vi "Write_parameter.vi"(8 "error in (no error)":errorcluster caption="entrée d'erreur (pas d'erreur)", 10 "Parameter":string, 11 "Class DIO en entrée":refnum<class "Class Instrument Ana.lvclass">) -> (0 "error out":errorcluster caption="sortie d'erreur", 3 "Class DIO en Sortie":refnum<class "Class Instrument Ana.lvclass">)   [LabVIEW 2020, in "Library Instrument & Equipement.lvlib" / "Library Instruments.lvlib" / "Class Instrument Ana.lvclass"]
uses:
  Class Instrument Ana.lvclass
  Ana/Class Ana (Default)/Class Ana (Default).lvclass
  JSON API/JSON Value/Set from JSON string.vi
  Instrument (Default)/Class Instrument (Default).lvclass
  JSON API/JSON Value/JSON Value.lvclass
  Class Instrument Ana.lvclass/Class Instrument Ana.ctl
  JSON API/Variant JSON/Variant JSON.lvlib
  JSON API/Get Polymorphic/JSON GetSet.lvlib
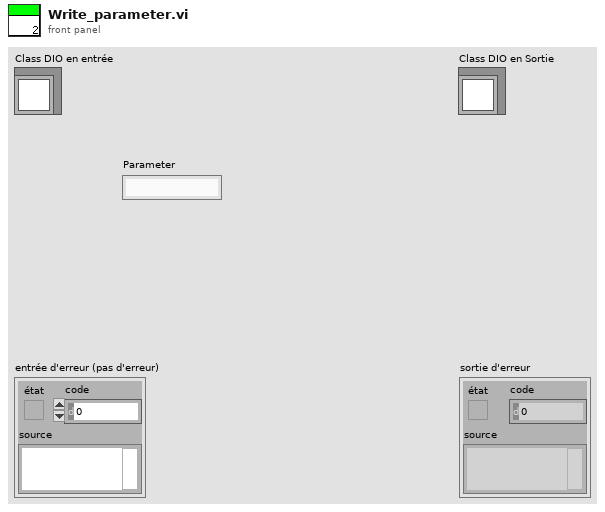
[diagram p1: front panel]
types:
  T1 = cluster{"Device_Com_Port":string, "Rate":u16, "Nb Sample":u16, "Voltage Max":dbl, "Voltage Min":dbl, "Input terminal Configuration":string, "Channel":u8[], "Continuous":bool, "Nb Data_To_Read":i16, "Class Ana":refnum<class "Class Ana (Default).lvclass">}
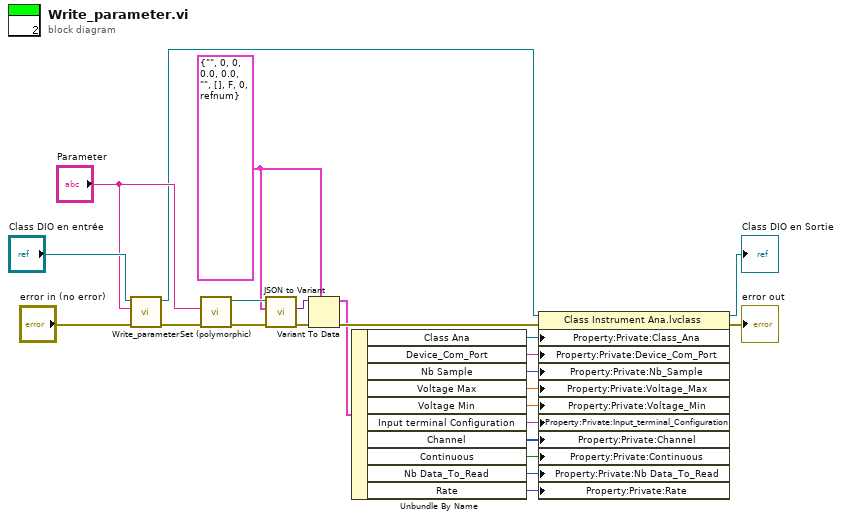
[diagram p0: block diagram]
diagram:
  w16 = T1 {"Device_Com_Port"="", "Rate"=0, "Nb Sample"=0, "Voltage Max"=0.0, "Voltage Min"=0.0, "Input terminal Configuration"="", "Channel"=[], "Continuous"=FALSE, "Nb Data_To_Read"=0, "Class Ana"=refnum} ("Parameter")
  n1 = call-parent "Write_parameter.vi"("error in (no error)"="error in (no error)", "Parameter"="Parameter", "Class Instrument (Default) en entrée"="Class DIO en entrée") -> ("error out"=w19:errorcluster, "Class Instrument (Default) en sortie"=w15:refnum<class "Class Instrument Ana.lvclass">)  [unwired: 7 in]
  n2 = call-poly "Set (polymorphic).vi"("error in (no error)"=w19, "JSON stream"="Parameter") -> ("error out"=w22:errorcluster, "JSON Value out"=w24:refnum<class "JSON Value.lvclass">)  [unwired: 7 in, 1 out]
  n3 = call "JSON to Variant.vi"("error in (no error)"=w22, "Variant (Data Type)"=w16, "JSON Value"=w24) -> ("error out"=w23:errorcluster, "Variant out"=w21:variant)  [unwired: 7 in]
  n4 = Variant To Data(error in=w23, type=w16, Variant=w21) -> (data=w1:T1, error out=w4:errorcluster)
  n5 = Unbundle By Name(w1) -> ("Class Ana"=w5:refnum<class "Class Ana (Default).lvclass">, "Device_Com_Port"=w6:string, "Nb Sample"=w7:u16, "Voltage Max"=w8:dbl, "Voltage Min"=w9:dbl, "Input terminal Configuration"=w10:string, "Channel"=w11:u8[], "Continuous"=w12:bool, "Nb Data_To_Read"=w13:i16, "Rate"=w14:u16)
  n6 = property class="Class Instrument Ana.lvclass"(reference=w15, error in=w4, "Property:Private:Class_Ana"=w5, "Property:Private:Device_Com_Port"=w6, "Property:Private:Nb_Sample"=w7, "Property:Private:Voltage_Max"=w8, "Property:Private:Voltage_Min"=w9, "Property:Private:Input_terminal_Configuration"=w10, "Property:Private:Channel"=w11, "Property:Private:Continuous"=w12, "Property:Private:Nb Data_To_Read"=w13, "Property:Private:Rate"=w14) -> (reference out=→"Class DIO en Sortie":refnum<class "Class Instrument Ana.lvclass">, error out=→"error out":errorcluster)
